vi "Example Loopback.vi"() -> ()   [LabVIEW 2010]
uses:
  C:/tf/play/labview/Tinkerforge.dll
  Tinkerforge.dll
panel:
  out "message":string
  in  "stop":bool
  in  "uid":string="amb"
  in  "port":i32=4223
  in  "host":string="localhost"
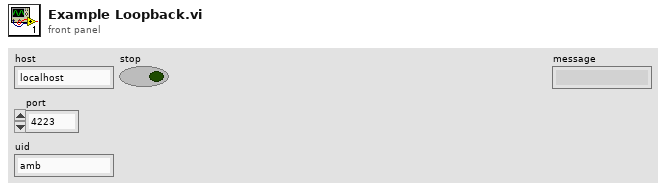
[diagram p1: front panel]
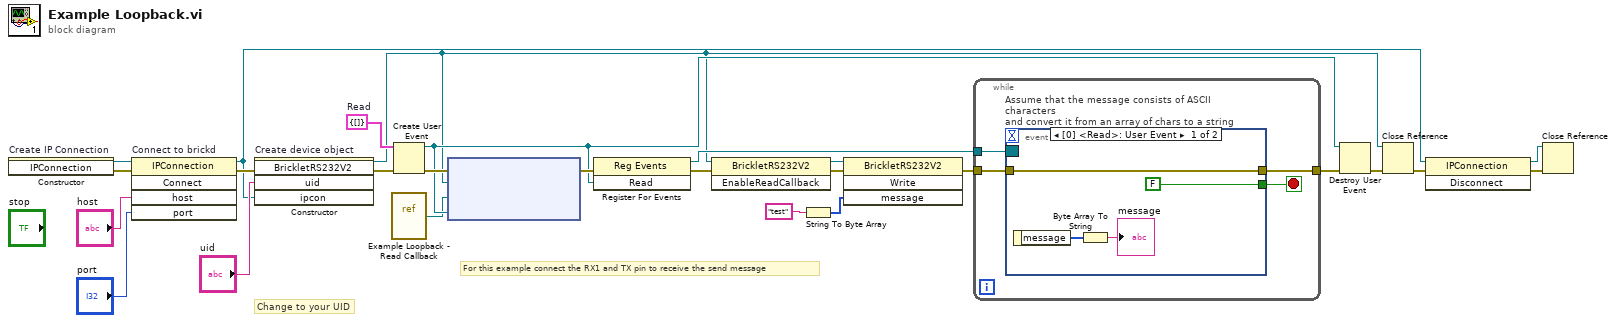
[diagram p0: block diagram]
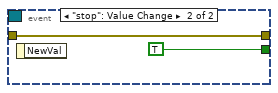
[diagram p2: hidden frame]
diagram:
  w10 = cluster{"message":u16[]} {"message"=[]}  # Read
  # "For this example connect the RX1 and TX pin to receive the send message"
  # "Change to your UID"
  n1 = constructor on="Create IP Connection" class="IPConnection"() -> (reference out=w26:refnum<k24>, error out=w11:errorcluster)  [unwired: 3 in, 1 out]
  n2 = invoke on="Connect to brickd" class="IPConnection" method="Connect"(reference=w26, error in=w11, "host"="host", "port"="port") -> (reference out=w19:refnum<k24>, error out=w22:errorcluster)  [unwired: 1 in, 3 out]
  n3 = constructor on="Create device object" class="BrickletRS232V2"(error in=w22, "uid"="uid", "ipcon"=w19) -> (reference out=w5:refnum<k24>, error out=w6:errorcluster)  [unwired: 2 in, 3 out]
  n4 = vi-ref "Example Loopback - Read Callback.vi"() -> ("vi reference"=w1:refnum<vi>)
  n5 = Create User Event(user event datatype=w10, error in=w6) -> (user event=w13:refnum<user-event>, error out=w17:errorcluster)
  n6 = node ("Register Event Callback")(w17, w5, w1, w13) -> (w16:errorcluster)  [unwired: 1 in, 1 out]
  n7 = register-events(error in=w16, w13) -> (reference out=w15:refnum<event-registration>, error out=w9:errorcluster)  [unwired: 1 in]
  n8 = invoke class="BrickletRS232V2" method="EnableReadCallback"(reference=w5, error in=w9) -> (reference out=w4:refnum<k24>, error out=w8:errorcluster)  [unwired: 1 in, 1 out]
  n9 = String To Byte Array(string="test") -> (unsigned byte array=w2:u8[])
  n10 = invoke class="BrickletRS232V2" method="Write"(reference=w4, error in=w8, "message"=w2) -> (error out=w7:errorcluster)  [unwired: 1 in, 3 out]
  n11 = while {
    tunnel: w15 -> [w30]
    tunnel: [w29] -> w14
    tunnel: w7 -> [w28]
    stop <- w27 stop-if-true
    n12 = event "Assume that the message consists of ASCII characters\nand convert it from an array of chars to a string" shown="[0] <Read>: User Event" {
      selector: w30 -> [_ _]
      dyn-events: _ -> [_ _]
      timeout: _ -> [_ _]
      tunnel: [w34 w35] -> w29
      tunnel: w28 -> [w34 w35]
      tunnel: [FALSE TRUE] -> w27
      event User Event {
        n13 = event-data() -> ("message"=w31:u16[])  [unwired: 1 in]
        n14 = Byte Array To String(unsigned byte array=w31) -> (string=→"message":string)
      }
      event "stop": Value Change {
        n15 = event-data() -> ()  [unwired: 1 in, 1 out]
      }
    }
  }
  n16 = Destroy User Event(user event=w13, error in=w14) -> (error out=w12:errorcluster)
  n17 = Close Reference(reference=w5, error in (no error)=w12) -> (error out=w21:errorcluster)
  n18 = invoke class="IPConnection" method="Disconnect"(reference=w19, error in=w21) -> (reference out=w18:refnum<k24>, error out=w20:errorcluster)  [unwired: 1 in, 1 out]
  n19 = Close Reference(reference=w18, error in (no error)=w20) -> ()  [unwired: 1 out]
